vi "Send Process Message.vi"(7 "Process ID":string, 8 "error in (no error)":errorcluster, 9 "Payload":variant, 10 "Command":string, 11 "Process in":refnum<class "Process.lvclass">) -> (0 "error out":errorcluster, 3 "Process out":refnum<class "Process.lvclass">)   [LabVIEW 2019, in "TimingDRV Engine.lvlib" / "Process.lvclass"]
uses:
  Process.lvclass
  Process.lvclass/Process.ctl
  TypeDefs/Message.ctl
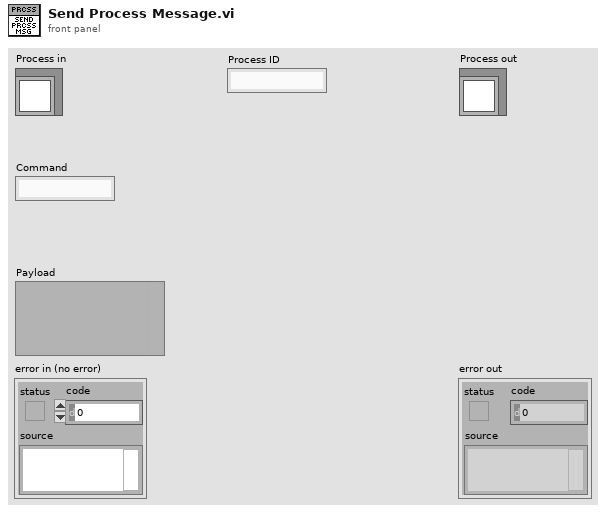
[diagram p1: front panel]
types:
  T1 = typedef "TimingDRV Engine.lvlib/Process.lvclass/Message.ctl" = cluster{"Command":string, "Payload":variant}
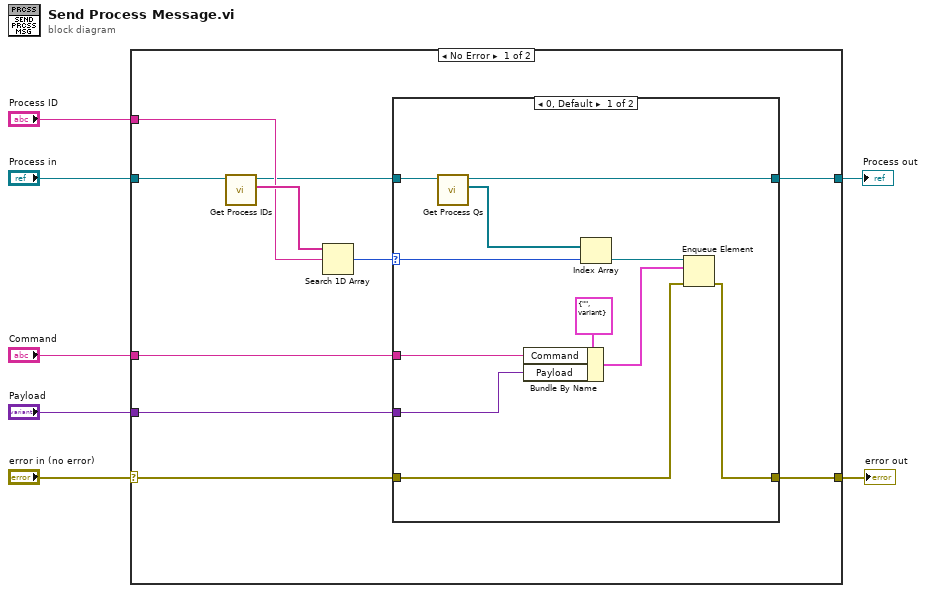
[diagram p0: block diagram]
diagram:
  n1 = case shown="No Error" "error in (no error)" {
    selector: "error in (no error)" -> [w9 w32]
    tunnel: [w8 w32] -> w6
    tunnel: [w10 w31] -> w4
    tunnel: "Process in" -> [w17 w31]
    tunnel: "Process ID" -> [w15 _]
    tunnel: "Command" -> [w12 _]
    tunnel: "Payload" -> [w11 _]
    frame No Error {
      n2 = call "Get Process IDs.vi"("Process in"=w17) -> ("Process IDs"=w16:string[], "Process out"=w14:refnum<class "Process.lvclass">)  [unwired: 9 in]
      n3 = Search 1D Array(1D array=w16, element=w15) -> (index of element=w13:i32)  [unwired: 1 in]
      n4 = case shown="0, Default" w13 {
        selector: w13 -> [w26 _]
        tunnel: w14 -> [w28 w30]
        tunnel: w12 -> [w22 _]
        tunnel: w11 -> [w21 _]
        tunnel: [w20 w30] -> w10
        tunnel: w9 -> [w19 w29]
        tunnel: [w18 w29] -> w8
        frame 0, Default {
          n5 = call "Get Process Qs.vi"("Process in"=w28) -> ("Process Qs"=w27:refnum<queue>[], "Process out"=w20:refnum<class "Process.lvclass">)  [unwired: 9 in]
          n6 = Bundle By Name(cluster=T1 {"Command"="", "Payload"=variant} ("element"), "Command"=w22, "Payload"=w21) -> (w23:T1)
          n7 = Index Array(array=w27, index=w26) -> (element=w25:refnum<queue>)
          n8 = Enqueue Element(queue=w25, element=w23, error in (no error)=w19) -> (error out=w18:errorcluster)  [unwired: 1 in, 2 out]
        }
        frame -1 {
        }
      }
    }
    frame Error {
    }
  }
  "error out" <- w6
  "Process out" <- w4
